vi "Calculate Distance.vi"(8 "error in (no error)":errorcluster, 11 "Pigeon in":refnum<class "Pigeon.lvclass">) -> (0 "error out":errorcluster, 2 "Distance [km]":i32, 3 "Pigeon out":refnum<class "Pigeon.lvclass">)   [LabVIEW 2019, in "Pigeon.lvclass"]
uses:
  Pigeon.lvclass
  C:/Users/Extensa/Desktop/Fabryka/Fabryka Rozwiazanie/Delivery/Delivery/Delivery.lvclass
  Delivery/Delivery.lvclass/Delivery.ctl
  Delivery/Delivery.lvclass
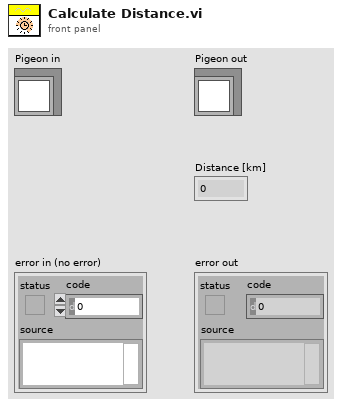
[diagram p1: front panel]
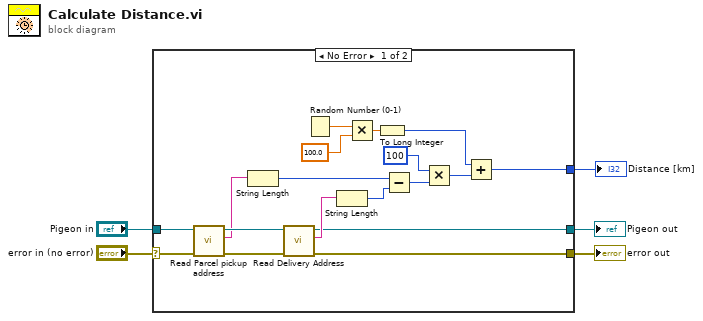
[diagram p0: block diagram]
diagram:
  n1 = case shown="No Error" "error in (no error)" {
    selector: "error in (no error)" -> [w23 w25]
    tunnel: [w7 w25] -> w4
    tunnel: [w8 w24] -> w2
    tunnel: "Pigeon in" -> [w22 w24]
    tunnel: [w6 _] -> w1
    frame No Error {
      n2 = call "Read Parcel pickup address.vi"("error in (no error)"=w23, "Delivery in"=w22) -> ("error out"=w20:errorcluster, "Parcel pickup address"=w19:string, "Delivery out"=w21:refnum<class "Pigeon.lvclass">)  [unwired: 7 in]
      n3 = String Length(string=w19) -> (length=w17:i32)
      n4 = call "Read Delivery Address.vi"("error in (no error)"=w20, "Delivery in"=w21) -> ("error out"=w7:errorcluster, "Delivery Address"=w18:string, "Delivery out"=w8:refnum<class "Pigeon.lvclass">)  [unwired: 7 in]
      n5 = Random Number (0-1)() -> (number: 0 to 1=w12:dbl)
      n6 = String Length(string=w18) -> (length=w16:i32)
      n7 = Multiply(x=w12, y=100.0) -> (x*y=w10:dbl)
      n8 = To Long Integer(number=w10) -> (32bit integer=w9:i32)
      n9 = Subtract(x=w17, y=w16) -> (x-y=w15:i32)
      n10 = Multiply(x=100, y=w15) -> (x*y=w13:i32)
      n11 = Add(x=w9, y=w13) -> (x+y=w6:i32)
    }
    frame Error {
    }
  }
  "error out" <- w4
  "Pigeon out" <- w2
  "Distance [km]" <- w1
